vi "Triangular Random.vi"(6 "seed":i32=-1, 7 "reset":bool, 8 "xmax":dbl=1.0, 9 "xmode":dbl=nan, 10 "xmin":dbl, 11 "samples":i32=128) -> (0 "error":i32, 3 "triangular random data":dbl[](array[numeric]))   [LabVIEW 2017, in "NI_Gmath.lvlib"]
doc: "Generates random values from a variate X, where X describes the selected distribution type. You must manually select the polymorphic instance to use."
uses:
  NI_Gmath.lvlib
panel:
  # "Triangular Random"
  # "NaN maps to \n(xmax-xmin)/2"
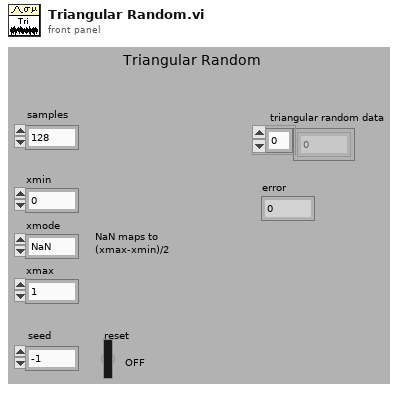
[diagram p1: front panel]
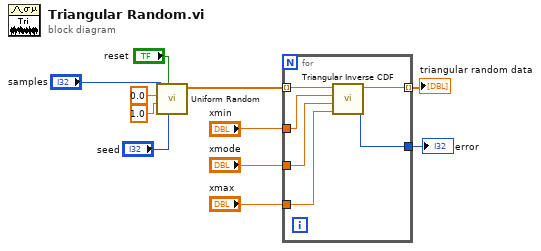
[diagram p0: block diagram]
diagram:
  n1 = call "Uniform Random.vi"("seed"="seed", "reset"="reset", "xmax"=1.0, "xmin"=0.0, "samples"="samples") -> ("uniform random data"=w3:dbl[])  [unwired: 5 in, 1 out]
  n2 = for {
    tunnel: "xmin" -> [w17]
    tunnel: [w16] -> w10 mode=indexing
    tunnel: [w15] -> w9
    tunnel: "xmode" -> [w14]
    tunnel: "xmax" -> [w13]
    tunnel: w3 -> [w12] mode=indexing
    n3 = call "Triangular Inverse CDF.vi"("xmax"=w13, "xmode"=w14, "xmin"=w17, "cdf(x)"=w12) -> ("error"=w15:i32, "x"=w16:dbl)  [unwired: 6 in]
  }
  "error" <- w9
  "triangular random data" <- w10
